vi "Hydra.vi"(7 "Hydra VISA Source":string, 11 "Hydra Write":string) -> (2 "OK?":bool, 3 "Response":string, 4 "error out":errorcluster)   [LabVIEW 2020, in "FBN_LATM.lvlib"]
uses:
  FBN_LATM.lvlib
  <vilib>/Instr/_visa.llb/VISA Configure Serial Port (Instr).vi
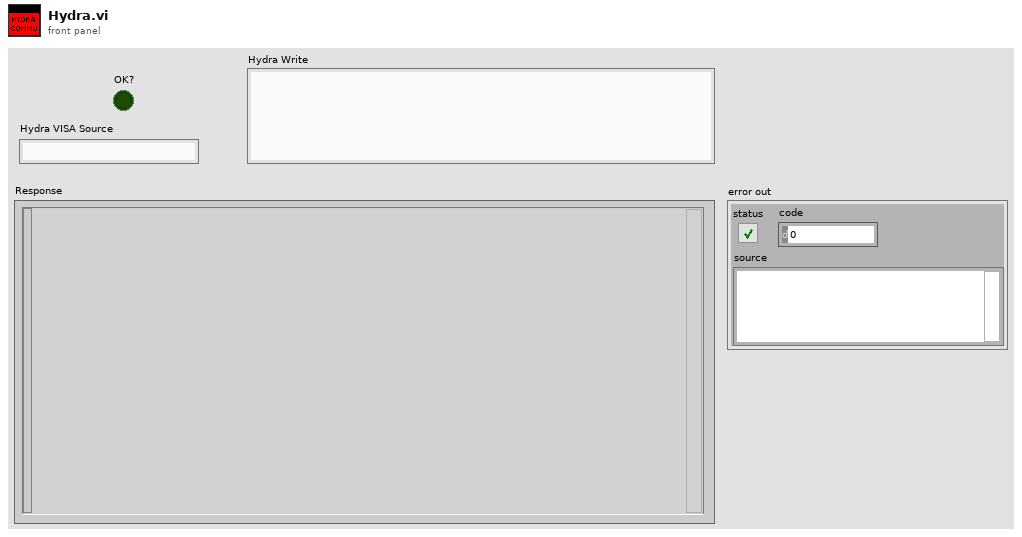
[diagram p1: front panel]
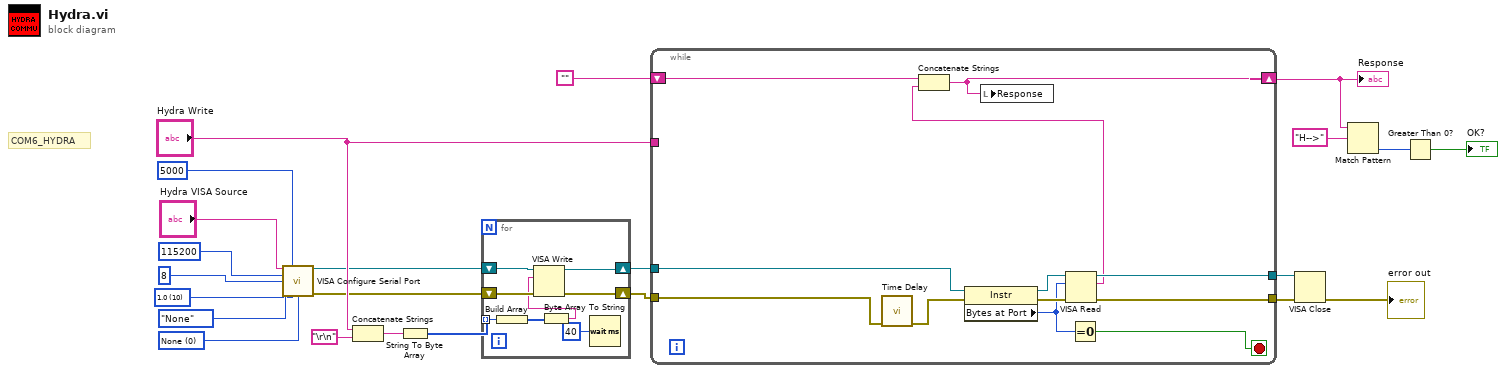
[diagram p0: block diagram]
diagram:
  w20 = u16 0 items=["None", "XON/XOFF", "RTS/CTS", "XON/XOFF & RTS/CTS", "DTR/DSR", "XON/XOFF & DTR/DSR"] ("flow control (0:none)")
  w21 = u16 10 items=["1.0"=10, "1.5"=15, "2.0"=20] ("stop bits (10: 1 bit)")
  # "COM6_HYDRA"
  n1 = call-poly "VISA Configure Serial Port"("VISA resource name"="Hydra VISA Source", "timeout (10sec)"=u32 5000, "baud rate (9600)"=u32 115200, "data bits (8)"=u16 8, "parity (0:none)"=enum16{"None", "Odd", "Even", "Mark", "Space"}."None", "stop bits (10: 1 bit)"=w21, "flow control (0:none)"=w20) -> ("VISA resource name out"=w8:refnum<visa-resource-name>, "error out"=w7:errorcluster)  [unwired: 2 in, 5 out]
  n2 = Concatenate Strings("Hydra Write", "\r\n") -> (w10:string)
  n3 = String To Byte Array(string=w10) -> (unsigned byte array=w9:u8[])
  n4 = for {
    shift-right: [w28] -> w6
    shift-left: w7 -> [w31]
    shift-right: [w29] -> w5
    shift-left: w8 -> [w30]
    tunnel: w9 -> [w27] mode=indexing
    n5 = Build Array(w27) -> (w26:u8[])
    n6 = Byte Array To String(unsigned byte array=w26) -> (string=w25:string)
    n7 = VISA Write(VISA resource name=w30, write buffer=w25, error in (no error)=w31) -> (VISA resource name out=w29:refnum<visa-resource-name>, error out=w28:errorcluster)  [unwired: 1 out]
    n8 = Wait (ms)(milliseconds to wait=u32 40) -> ()  [unwired: 1 out]
  }
  n9 = while {
    shift-right: [w37] -> w2
    shift-left: "" -> [w41]
    tunnel: [w39] -> w16
    tunnel: [w38] -> w15
    tunnel: w6 -> [w35]
    tunnel: w5 -> [w34]
    tunnel: "Hydra Write" -> [_]
    stop <- w32 stop-if-true
    n10 = call "Time Delay"("error in (no error)"=w35) -> ("error out"=w40:errorcluster)  [unwired: 10 in]
    n11 = property class="Instr"(reference=w34, error in=w40) -> (reference out=w43:refnum<visa-resource-name>, error out=w42:errorcluster, "Bytes at Port"=w33:u32)
    n12 = VISA Read(VISA resource name=w43, byte count=w33, error in (no error)=w42) -> (VISA resource name out=w38:refnum<visa-resource-name>, read buffer=w36:string, error out=w39:errorcluster)  [unwired: 1 out]
    n13 = Concatenate Strings(w41, w36) -> (w37:string)
    n14 = local write "Response"(w37) -> ()
    n15 = Equal To 0?(x=w33) -> (x = 0?=w32:bool)
  }
  "Response" <- w2
  n16 = VISA Close(VISA resource name=w15, error in (no error)=w16) -> (error out=→"error out":errorcluster)
  n17 = Match Pattern(string=w2, regular expression="H-->" ("replace string (\"\")")) -> (offset past match=w3:i32)  [unwired: 1 in, 3 out]
  n18 = Greater Than 0?(x=w3) -> (x > 0?=→"OK?":bool)
